vi "LCfiletransfer(SubVI).vi"(8 "error in (no error)":errorcluster, 9 "Source Filename":string, 11 "VISA Refnum in":refnum<visa-resource-name>) -> (0 "error out":errorcluster, 2 "File data":string, 3 "VISA Refnum out":refnum<visa-resource-name>)   [LabVIEW 2018]
uses:
  <instrlib>/LeCroy Wave Series/LeCroy Wave Series.lvlib
panel:
  in  "file path (use dialog)":path
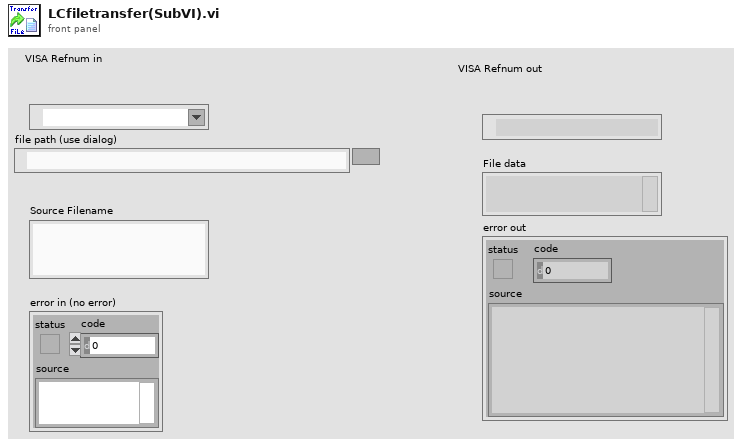
[diagram p1: front panel]
types:
  T1 = enum16{"open", "replace", "create", "open or create", "replace or create", "replace or create with confirmation"}
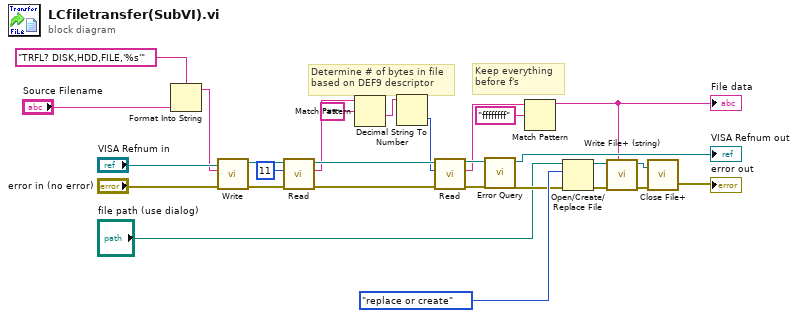
[diagram p0: block diagram]
diagram:
  # "Keep everything \nbefore f's"
  # "Determine # of bytes in file\nbased on DEF9 descriptor"
  n1 = Format Into String(format string="TRFL? DISK,HDD,FILE,'%s'" ("initial string"), "Source Filename") -> (resulting string=w23:string)  [unwired: 2 in, 1 out]
  n2 = call <instrlib>:"Write.vi"("error in (no error)"="error in (no error)", "Write Buffer"=w23, "VISA resource name"="VISA Refnum in") -> ("error out"=w19:errorcluster, "VISA resource name out"=w22:refnum<visa-resource-name>)  [unwired: 7 in]
  n3 = call <instrlib>:"Read.vi"("error in (no error)"=w19, "Byte Count"=u32 11, "VISA resource name"=w22) -> ("error out"=w18:errorcluster, "Read Buffer"=w16:string, "VISA resource name out"=w21:refnum<visa-resource-name>)  [unwired: 5 in, 1 out]
  n4 = Match Pattern(string=w16, regular expression="#9") -> (after substring=w14:string)  [unwired: 1 in, 3 out]
  n5 = Decimal String To Number(string=w14) -> (number=w13:i32)  [unwired: 2 in, 1 out]
  n6 = call <instrlib>:"Read.vi"("error in (no error)"=w18, "Byte Count"=w13, "VISA resource name"=w21) -> ("error out"=w8:errorcluster, "Read Buffer"=w11:string, "VISA resource name out"=w20:refnum<visa-resource-name>)  [unwired: 5 in, 1 out]
  n7 = call <instrlib>:"Error Query.vi"("error in (no error)"=w8, "VISA resource name"=w20) -> ("error out"=w7:errorcluster, "VISA resource name out"=→"VISA Refnum out":refnum<visa-resource-name>)  [unwired: 6 in, 2 out]
  n8 = Match Pattern(string=w11, regular expression="ffffffff") -> (before substring=w2:string)  [unwired: 1 in, 3 out]
  "File data" <- w2
  n9 = Open/Create/Replace File(file path (use dialog)="file path (use dialog)", error in=w7, operation (0:open)=T1."replace or create") -> (refnum out=w6:refnum<file>, error out=w10:errorcluster)  [unwired: 3 in, 1 out]
  n10 = call <vilib>:"Write File+ (string).vi"("string"=w2, "error in (no error)"=w10, "refnum"=w6) -> ("error out"=w9:errorcluster, "dup refnum"=w5:refnum<file>)  [unwired: 4 in, 1 out]
  n11 = call <vilib>:"Close File+.vi"("error in (no error)"=w9, "refnum"=w5) -> ("error out"=→"error out":errorcluster)  [unwired: 3 in, 2 out]
